vi "S_WriteClassAttribute.vi"(0 "reference in":refnum<class "SubTemplate_4x4x4.lvclass">, 5 "error in (no error)":errorcluster) -> (14 "reference out":refnum<class "SubTemplate_4x4x4.lvclass">, 19 "error out":errorcluster)   [LabVIEW 2020]
uses:
  SubTemplate_4x4x4.lvclass
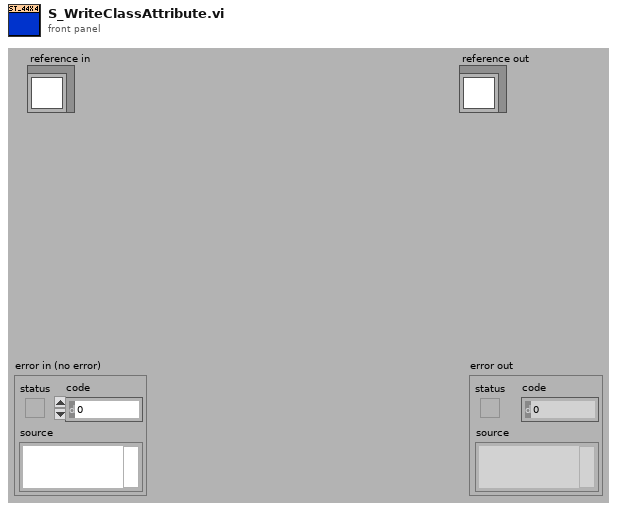
[diagram p1: front panel]
types:
  T1 = typedef "SubTemplate_4x4x4.lvclass/ClassAttributes.ctl" = cluster{"Base class":T2}
  T2 = typedef "BaseTemplate_4x4x4.lvclass/ClassAttributes.ctl" = cluster{"classAttribute1":bool}
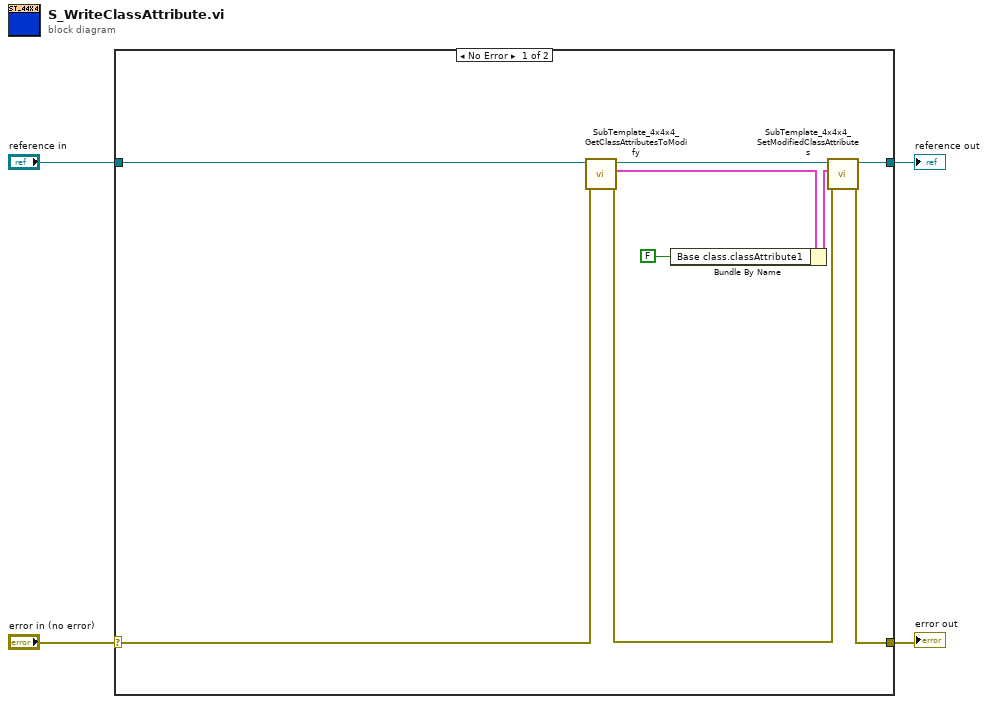
[diagram p0: block diagram]
diagram:
  n1 = case shown="No Error" "error in (no error)" {
    selector: "error in (no error)" -> [w7 w15]
    tunnel: [w10 w15] -> w3
    tunnel: [w9 w14] -> w1
    tunnel: "reference in" -> [w6 w14]
    frame No Error {
      n2 = call "SubTemplate_4x4x4_GetClassAttributesToModify.vi"("error in (no error)"=w7, "reference in"=w6) -> ("error out"=w8:errorcluster, "Class attributes"=w13:T1, "reference out"=w11:refnum<class "SubTemplate_4x4x4.lvclass">)  [unwired: 6 in, 1 out]
      n3 = Bundle By Name(cluster=w13, "Base class.classAttribute1"=FALSE) -> (w12:T1)
      n4 = call "SubTemplate_4x4x4_SetModifiedClassAttributes.vi"("error in (no error)"=w8, "Class attributes"=w12, "reference in"=w11) -> ("error out"=w10:errorcluster, "reference out"=w9:refnum<class "SubTemplate_4x4x4.lvclass">)  [unwired: 7 in]
    }
    frame Error {
    }
  }
  "error out" <- w3
  "reference out" <- w1
